vi "Read Type.vi"(8 "Error In":errorcluster, 11 "Tag In":refnum<class "Tag.lvclass">) -> (0 "Error Out":errorcluster, 2 "Type":T1, 3 "Tag Out":refnum<class "Tag.lvclass">)   [LabVIEW 2017, in "Mustache.lvlib" / "Tokens.lvlib" / "Tag.lvclass"]
uses:
  Tag.lvclass
  Controls/Types.ctl
  Tag.lvclass/Tag.ctl
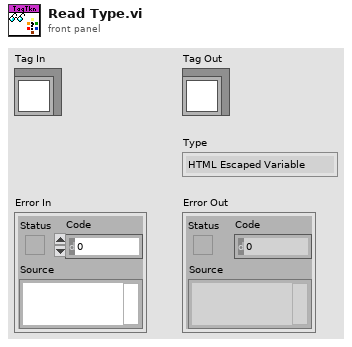
[diagram p1: front panel]
types:
  T1 = typedef "Mustache.lvlib/Tokens.lvlib/Tag.lvclass/Types.ctl" = enum16{"HTML Escaped Variable", "HTML Unescaped Variable", "Unescaped Variable", "Begin Section", "Invert Section", "End Section", "Comment", "Partial", "Set Delimiter"}
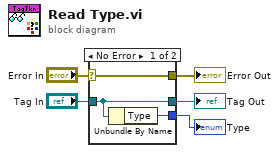
[diagram p0: block diagram]
diagram:
  n1 = case shown="No Error" "Error In" {
    selector: "Error In" -> [w8 w9]
    tunnel: [w8 w9] -> w4
    tunnel: [w7 w10] -> w2
    tunnel: "Tag In" -> [w7 w10]
    tunnel: [w6 _] -> w1
    frame No Error {
      n2 = Unbundle By Name(w7) -> ("Type"=w6:T1)
    }
    frame Error {
    }
  }
  "Error Out" <- w4
  "Tag Out" <- w2
  "Type" <- w1
